vi "Do.vi"(8 "error in (no error)":errorcluster, 10 "Actor in":refnum<class "Actor.lvclass">, 11 "Remote Island Msg":refnum<class "Remote Island Msg.lvclass">) -> (0 "error out":errorcluster, 2 "Actor out":refnum<class "Actor.lvclass">)   [LabVIEW 2018, in "EMS User Interface Actor.lvlib" / "Remote Island Msg.lvclass"]
doc: "This VI delivers the message to the actor by calling the appropriate method(s) on the actor."
uses:
  Remote Island Msg.lvclass
  C:/Users/Administrator/Desktop/2018LabVIEW EMS/Remote Operation/Remote Operation Abstract Messages/Island Microgrid Msg/Island Microgrid Msg.lvclass
  <vilib>/ActorFramework/Actor/Actor.lvclass
  EMS User Interface/EMS User Interface.lvclass
  C:/Program Files (x86)/National Instruments/LabVIEW 2018/vi.lib/ActorFramework/Actor/Actor.lvclass
  Remote Operation/Remote Operation Abstract Messages/Island Microgrid Msg/Island Microgrid Msg.lvclass/Island Microgrid Msg.ctl
  Remote Operation/Remote Operation Abstract Messages/Island Microgrid Msg/Island Microgrid Msg.lvclass
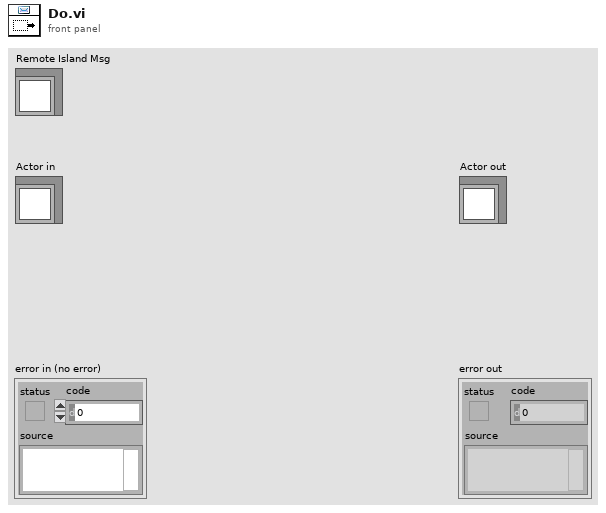
[diagram p1: front panel]
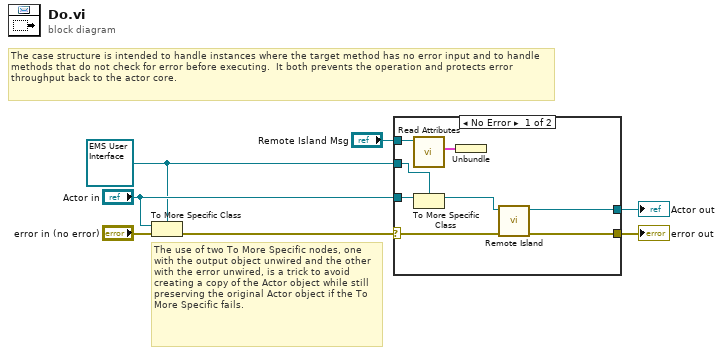
[diagram p0: block diagram]
diagram:
  w2 = refnum<class "EMS User Interface.lvclass"> refnum ("Actor in")
  # "The use of two To More Specific nodes, one with the output object unwired and the other with the error unwired, is a trick to avoid creating a copy of the Actor object while still preserving the original Actor object if the To More Specific fails."
  # "The case structure is intended to handle instances where the target method has no error input and to handle methods that do not check for error before executing.  It both prevents the operation and protects error throughput back to the actor core."
  n1 = To More Specific Class(target class=w2, reference="Actor in", error in="error in (no error)") -> (error out=w6:errorcluster)  [unwired: 1 out]
  n2 = case shown="No Error" w6 {
    selector: w6 -> [w13 w17]
    tunnel: [w15 w17] -> w5
    tunnel: [w14 w16] -> w4
    tunnel: "Actor in" -> [w12 w16]
    tunnel: w2 -> [w11 _]
    tunnel: "Remote Island Msg" -> [w8 _]
    frame No Error {
      n3 = call "Read Attributes.vi"("Island Microgrid Msg"=w8) -> ("Payload"=w9:cluster{"Data":variant})  [unwired: 10 in]
      n4 = To More Specific Class(target class=w11, reference=w12) -> (specific class reference=w10:refnum<class "EMS User Interface.lvclass">)  [unwired: 1 in, 1 out]
      n5 = Unbundle(w9) -> ()  [unwired: 1 out]
      n6 = call "Remote Island.vi"("error in"=w13, "Master Controller in"=w10) -> ("error out"=w15:errorcluster, "Master Controller out"=w14:refnum<class "EMS User Interface.lvclass">)  [unwired: 8 in]
    }
    frame Error {
      # "If type check fails, pass the original object out again."
    }
  }
  "error out" <- w5
  "Actor out" <- w4
